vi "Setup Local Resources.vi"(8 "error in (no error)":errorcluster, 11 "1553 SubComponent in":refnum<class "1553 SubComponent.lvclass">) -> (0 "error out":errorcluster, 3 "1553 SubComponent out":refnum<class "1553 SubComponent.lvclass">)   [LabVIEW 2020, in "BCI-1553 API.lvlib" / "1553 SubComponent.lvclass"]
doc: "Initializes the various parameter and addres tables in class data. All child classes should call this at some point early in their initialization code."
uses:
  1553 SubComponent.lvclass
  Dependencies/Registry/Registry.lvclass/Registry.ctl
  1553 SubComponent.lvclass/1553 SubComponent.ctl
  Dependencies/Registry/Registry.lvclass
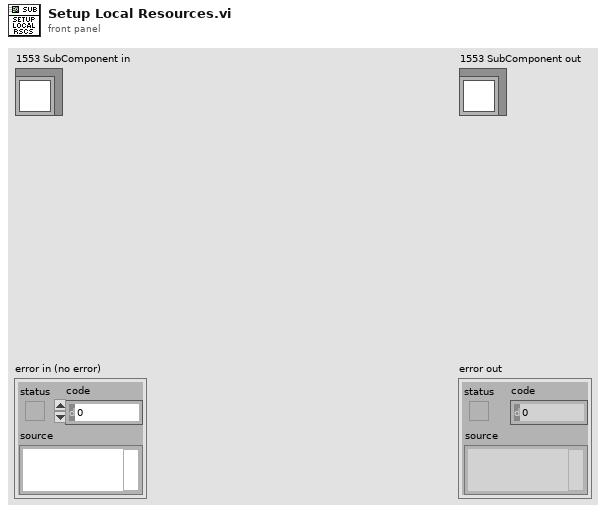
[diagram p1: front panel]
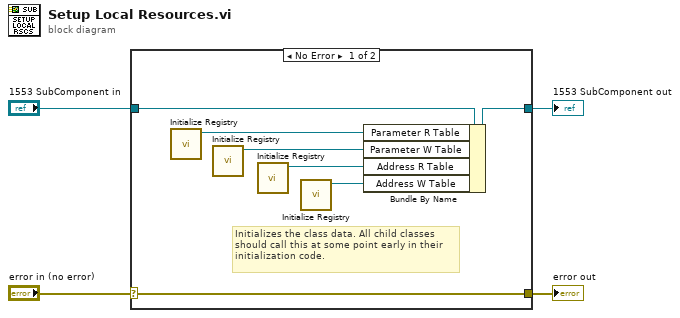
[diagram p0: block diagram]
diagram:
  n1 = case shown="No Error" "error in (no error)" {
    selector: "error in (no error)" -> [w11 w13]
    tunnel: [w11 w13] -> w3
    tunnel: [w9 w12] -> w1
    tunnel: "1553 SubComponent in" -> [w10 w12]
    frame No Error {
      # "Initializes the class data. All child classes\nshould call this at some point early in their\ninitialization code."
      n2 = call "Initialize Registry.vi"() -> ("Registry out"=w8:refnum<class "Registry.lvclass">)  [unwired: 10 in, 1 out]
      n3 = call "Initialize Registry.vi"() -> ("Registry out"=w7:refnum<class "Registry.lvclass">)  [unwired: 10 in, 1 out]
      n4 = call "Initialize Registry.vi"() -> ("Registry out"=w6:refnum<class "Registry.lvclass">)  [unwired: 10 in, 1 out]
      n5 = call "Initialize Registry.vi"() -> ("Registry out"=w5:refnum<class "Registry.lvclass">)  [unwired: 10 in, 1 out]
      n6 = Bundle By Name(cluster=w10, "Parameter R Table"=w8, "Parameter W Table"=w7, "Address R Table"=w6, "Address W Table"=w5) -> (w9:refnum<class "1553 SubComponent.lvclass">)
    }
    frame Error {
    }
  }
  "error out" <- w3
  "1553 SubComponent out" <- w1
